vi "gentec-M-Link.Current Measurement.vi"(0 "VISA resource In":refnum<visa-resource-name>, 2 "Measurement":T2 items=["other Mode", "Energymode"], 5 "error in (no error)":errorcluster) -> (8 "Out":bool, 10 "New Data":bool, 11 "Data Read":string, 12 "No Probe":bool, 13 "Read Timeout":bool, 14 "VISA resource Out":refnum<visa-resource-name>, 15 "Range":T1 items=["1f", "3f", "10f", "30f", "100f", "300f", "1p", "3p", "10p", "30p", "100p", "300p", "1n", "3n", "10n", "30n", "100n", "300n", "1u", "3u", "10u", "30u", "100u", "300u", "1m", "3m", "10m", "30m", "100m", "300m", "1", "3", "10", "30", "100", "300", "1K", "3K", "10K", "30K", "100K", "300K", "1M", "3M", "10M", "30M", "100M", "300M"], 16 "ADC Counts":u16, 17 "Pulse Period Counts":u32, 19 "error out":errorcluster)   [LabVIEW 2014, in "gentec-M-Link - Driver.lvlib"]
doc: "Data to write: cur0 or cur1\n\nQuery only. Returns the current measurement. The argument is 1 for Energy Heads, Radiometric Heads, or Radiometer heads in Energy mode, and 0 for all others. Data is sent as certain hexadecimal data string."
uses:
  gentec-M-Link - Driver.lvlib
  Type Defs/gentec-M-Link.Measurement Mode.ctl
  Type Defs/gentec-M-Link.Range.ctl
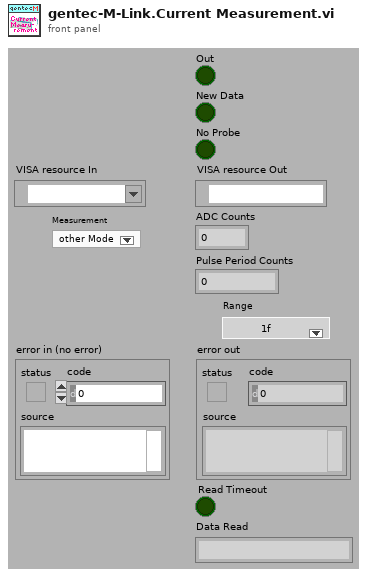
[diagram p1: front panel]
types:
  T1 = typedef "gentec-M-Link - Driver.lvlib/gentec-M-Link.Range.ctl" = u16
  T2 = typedef "gentec-M-Link - Driver.lvlib/gentec-M-Link.Measurement Mode.ctl" = u16
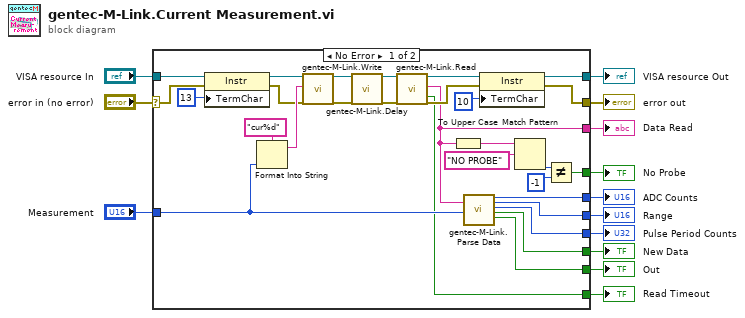
[diagram p0: block diagram]
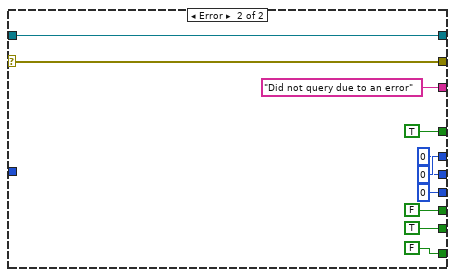
[diagram p2: hidden frame]
diagram:
  n1 = case shown="No Error" "error in (no error)" {
    selector: "error in (no error)" -> [w29 w52]
    tunnel: [w22 w52] -> w12
    tunnel: "VISA resource In" -> [w30 w51]
    tunnel: "Measurement" -> [w20 _]
    tunnel: [w31 u32 0 ("Pulse Period Counts")] -> w9
    tunnel: [w35 i16 0 ("ADC Counts")] -> w8
    tunnel: [w34 TRUE] -> w7
    tunnel: [w17 u16 0 ("Range")] -> w6
    tunnel: [w33 FALSE ("new SSE")] -> w5
    tunnel: [w32 TRUE ("OUT")] -> w4
    tunnel: [w24 w51] -> w3
    tunnel: [w19 "Did not query due to an error" ("Data Read")] -> w2
    tunnel: [w18 FALSE ("Timeout")] -> w1
    frame No Error {
      n2 = property class="Instr"(reference=w30, error in=w29, "TermChar"=u8 13 ("Message Based Settings:Termination Character")) -> (reference out=w27:refnum<visa-resource-name>, error out=w28:errorcluster)
      n3 = Format Into String(format string="cur%d" ("Data To Write"), w20) -> (resulting string=w41:string)  [unwired: 2 in, 1 out]
      n4 = call "gentec-M-Link.Write.vi"("VISA resource (In)"=w27, "Data To Write"=w41, "error in (no error)"=w28) -> ("VISA resource (Out)"=w15:refnum<visa-resource-name>, "error out"=w36:errorcluster)  [unwired: 14 in, 1 out]
      n5 = call "gentec-M-Link.Delay.vi"("VISA resource In"=w15, "error in (no error)"=w36) -> ("VISA resource Out"=w14:refnum<visa-resource-name>, "error out"=w16:errorcluster)  [unwired: 16 in]
      n6 = call "gentec-M-Link.Read.vi"("VISA resource (In)"=w14, "error in (no error)"=w16) -> ("VISA resource (Out)"=w25:refnum<visa-resource-name>, "Data Read"=w19:string, "Read Timeout"=w18:bool, "error out"=w23:errorcluster)  [unwired: 13 in, 1 out]
      n7 = To Upper Case(1:w19) -> (0:w40:string)
      n8 = call "gentec-M-Link.Parse Data.vi"("Data Bytes"=w19, "Measurement"=w20) -> ("ADC Counts"=w35:u16, "Range"=w17:T1, "Pulse Period Counts"=w31:u32, "new SSE"=w33:bool, "Out"=w32:bool)  [unwired: 13 in]
      n9 = property class="Instr"(reference=w25, error in=w23, "TermChar"=u8 10 ("Message Based Settings:Termination Character")) -> (reference out=w24:refnum<visa-resource-name>, error out=w22:errorcluster)
      n10 = Match Pattern(string=w40, regular expression="NO PROBE") -> (offset past match=w38:i32)  [unwired: 1 in, 3 out]
      n11 = Not Equal?(x=w38, y=-1) -> (x != y?=w34:bool)
    }
    frame Error {
    }
  }
  "error out" <- w12
  "Pulse Period Counts" <- w9
  "ADC Counts" <- w8
  "No Probe" <- w7
  "Range" <- w6
  "New Data" <- w5
  "Out" <- w4
  "VISA resource Out" <- w3
  "Data Read" <- w2
  "Read Timeout" <- w1
